vi "Ref Index.vi"(8 "error in":errorcluster, 10 "Label":string, 11 "Map Out":map{string, refnum<vi>}(c390)) -> (0 "error out":errorcluster, 2 "key not found?":bool, 3 "value":refnum<vi>)   [LabVIEW 2020]
uses:
  <vilib>/Utility/error.llb/Error Cluster From Error Code.vi
  <vilib>/ErrorRing/Error Ring.xnode
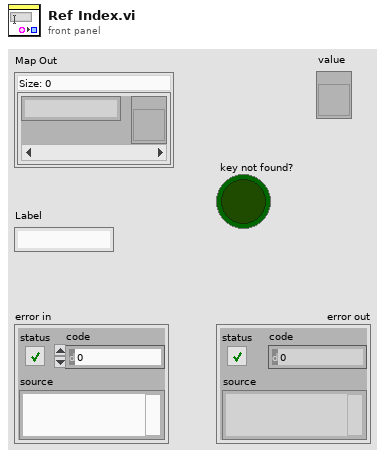
[diagram p1: front panel]
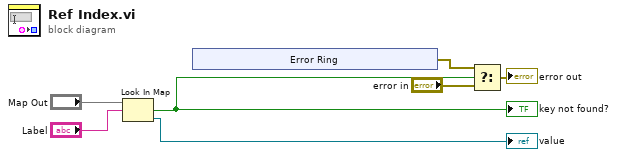
[diagram p0: block diagram]
diagram:
  n1 = Look In Map(map="Map Out", key="Label") -> (key not found?=w2:bool, value=→"value":refnum<vi>)  [unwired: 1 in]
  "key not found?" <- w2
  n2 = xnode "Error Ring"() -> ("error out"=w4:errorcluster)
  n3 = Select(t=w4, s=w2, f="error in") -> (s? t:f=→"error out":errorcluster)
